vi "Session Initialization Parameters from Resource Name.vi"(11 "resource name":string) -> (3 "session initialization parameters":T1)   [LabVIEW 2020, in "MeasurementServerTests.lvlib"]
uses:
  MeasurementServerTests.lvlib
  Runtime/Sessions/Instrument/ISession Factory/Session Initialization Parameters.ctl
  Runtime/Sessions/Instrument/ISession Factory/ISession Factory.lvclass
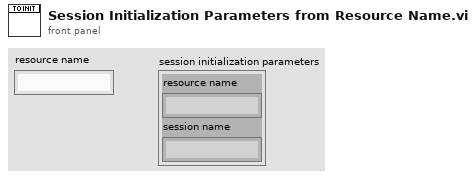
[diagram p1: front panel]
types:
  T1 = typedef "NI Session Management Instrument.lvlib/ISession Factory.lvclass/Session Initialization Parameters.ctl" = cluster{"resource name":string, "session name":string}
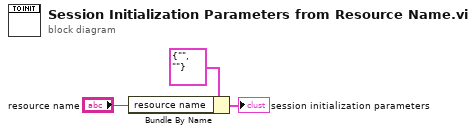
[diagram p0: block diagram]
diagram:
  n1 = Bundle By Name(cluster=T1 {"resource name"="", "session name"=""} ("session initialization details"), "resource name"="resource name") -> (→"session initialization parameters":T1)
